vi "SDSU_ReadDACS_orig.vi"(7 "fd":i32, 8 "error in (no error)":errorcluster, 9 "argument":string, 10 "action":T1(ring), 11 "file path":path=path "/home/arcconfig/DHE_DACS.cfg") -> (0 "error out":errorcluster, 1 "response":string, 2 "Table":string[][](table), 3 "file path out":path=path "/home/ArcVIEW/ConfigFiles/PI_laboratory.cfg", 5 "index":i32, 6 "fd out":i32)   [LabVIEW 2016]
panel:
  out "resolutions":string[][](array[string])
  in  "current index":u8=6
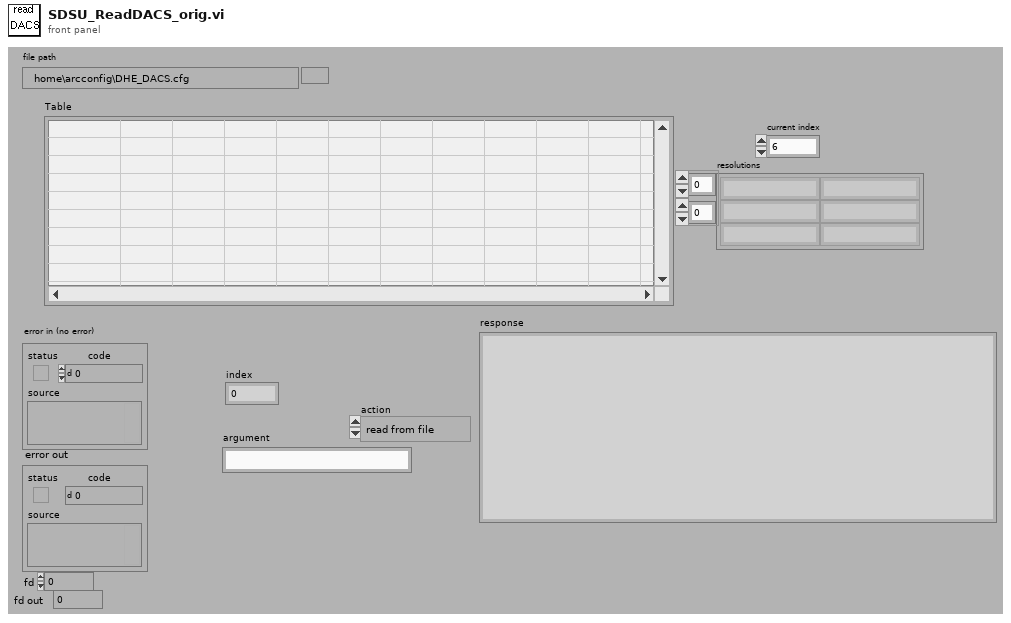
[diagram p1: front panel]
types:
  T1 = enum16{"read from file", "find", "set", "set_to_default", "get all"}
  T2 = typedef "DatabaseHand_RefNum.ctl" = refnum<vi>
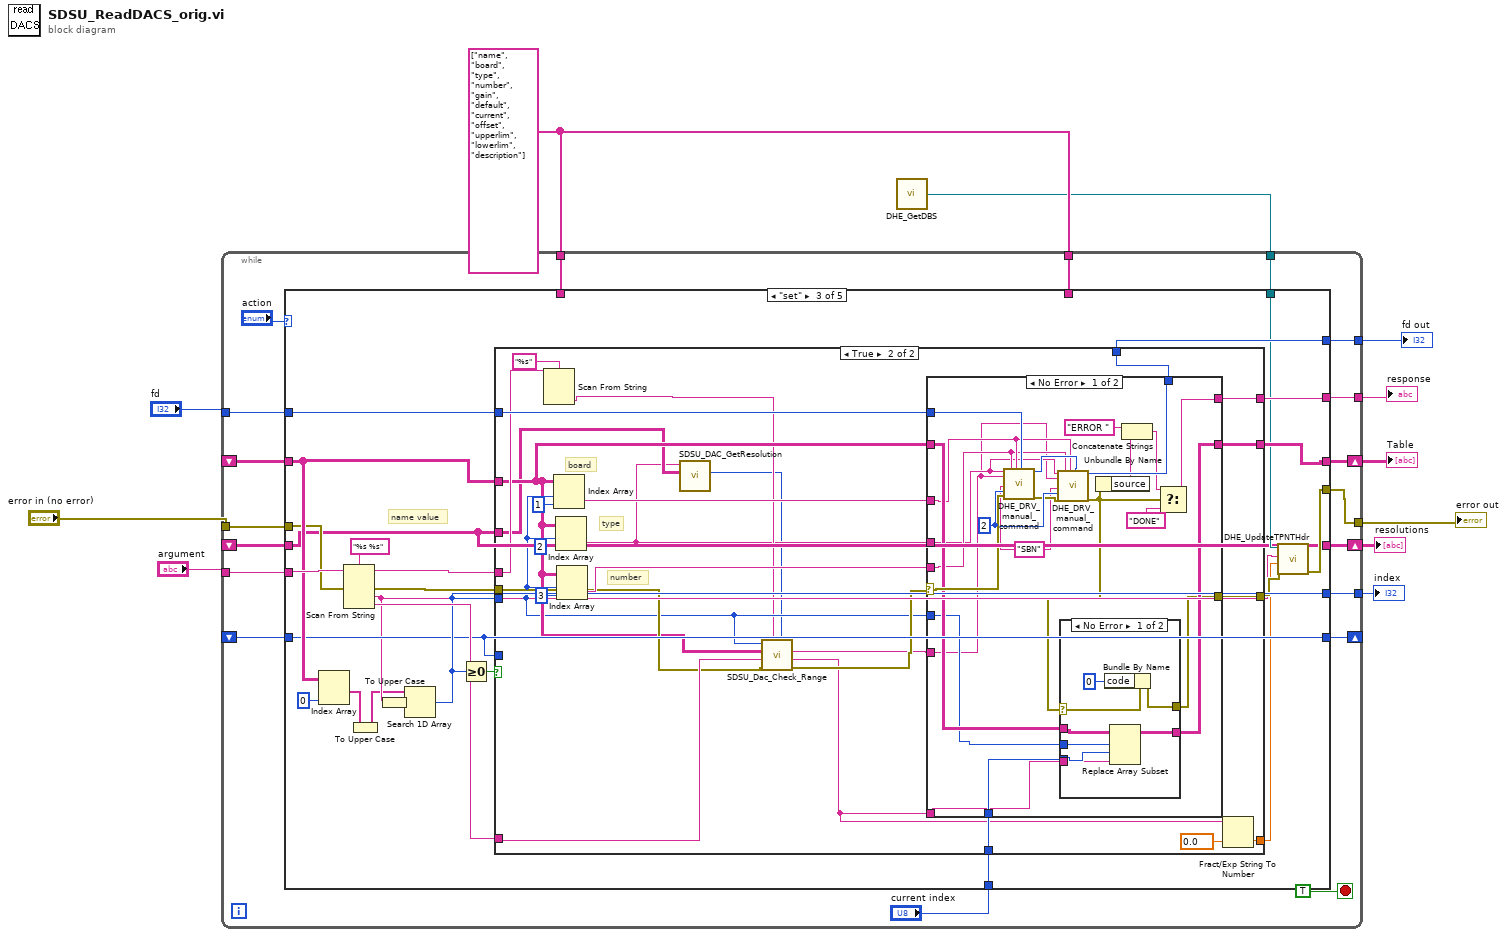
[diagram p0: block diagram]
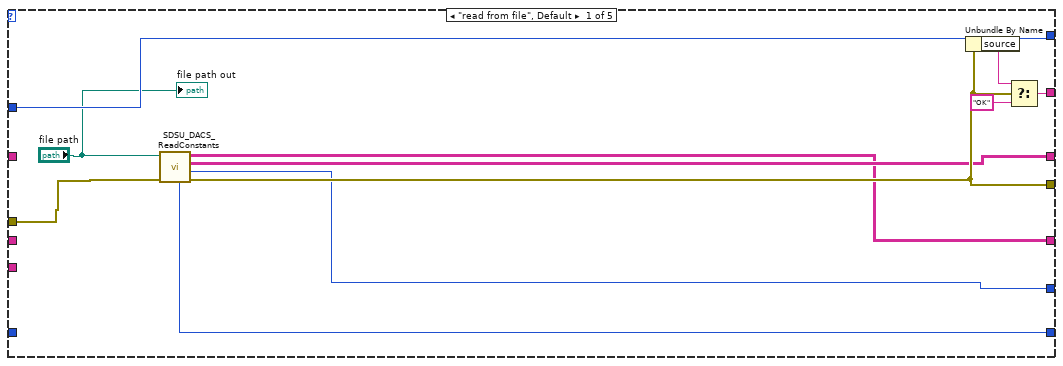
[diagram p2: hidden frame]
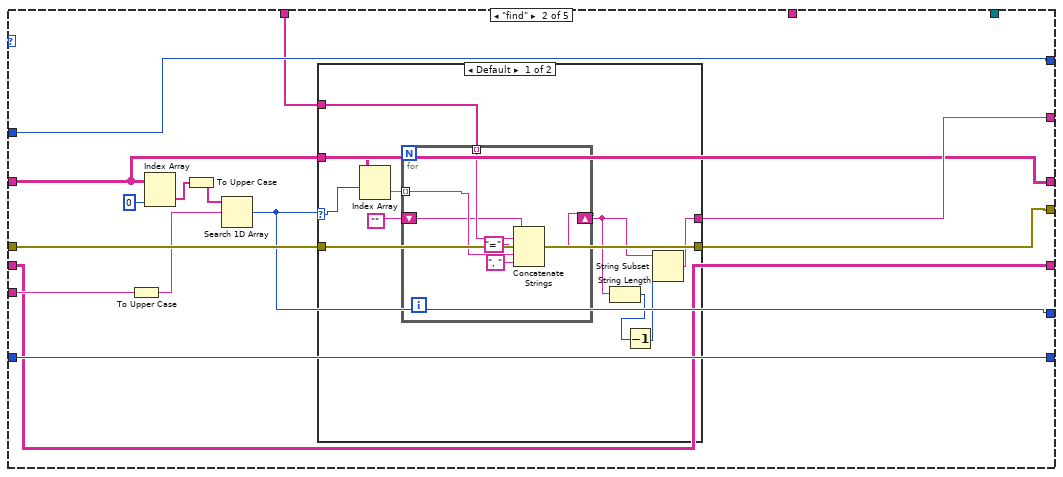
[diagram p3: hidden frame]
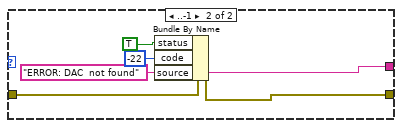
[diagram p4: hidden frame]
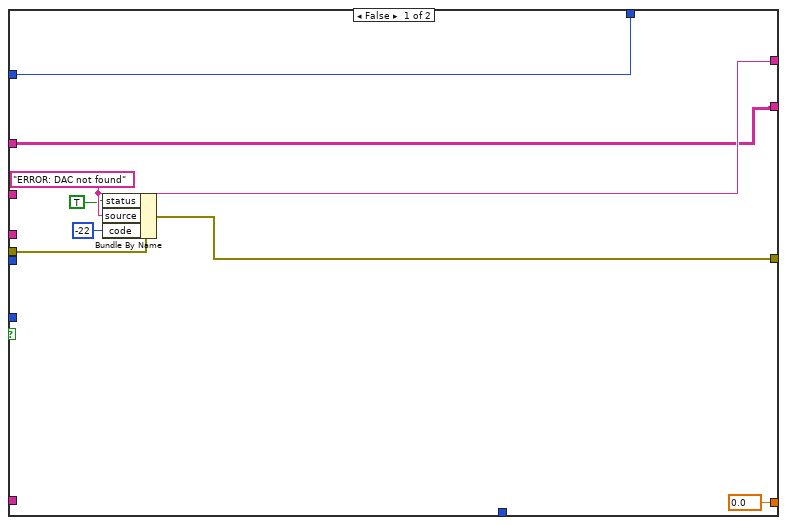
[diagram p5: hidden frame]
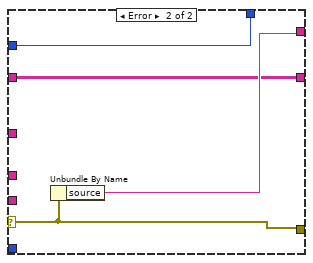
[diagram p7: hidden frame]
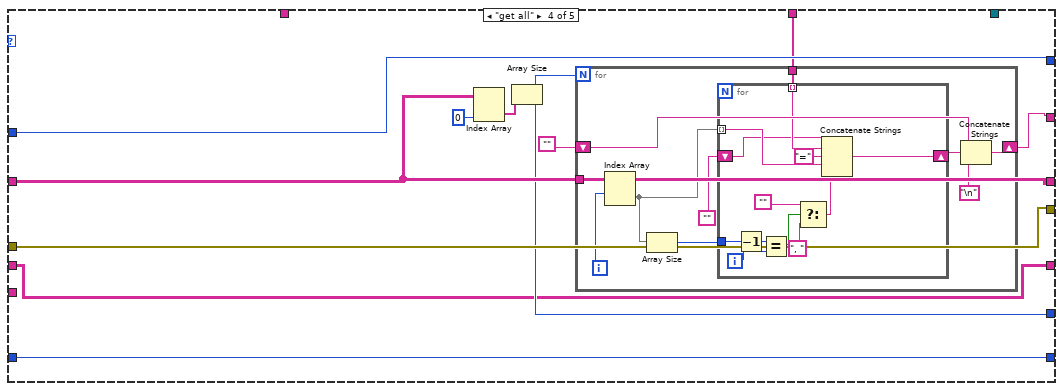
[diagram p8: hidden frame]
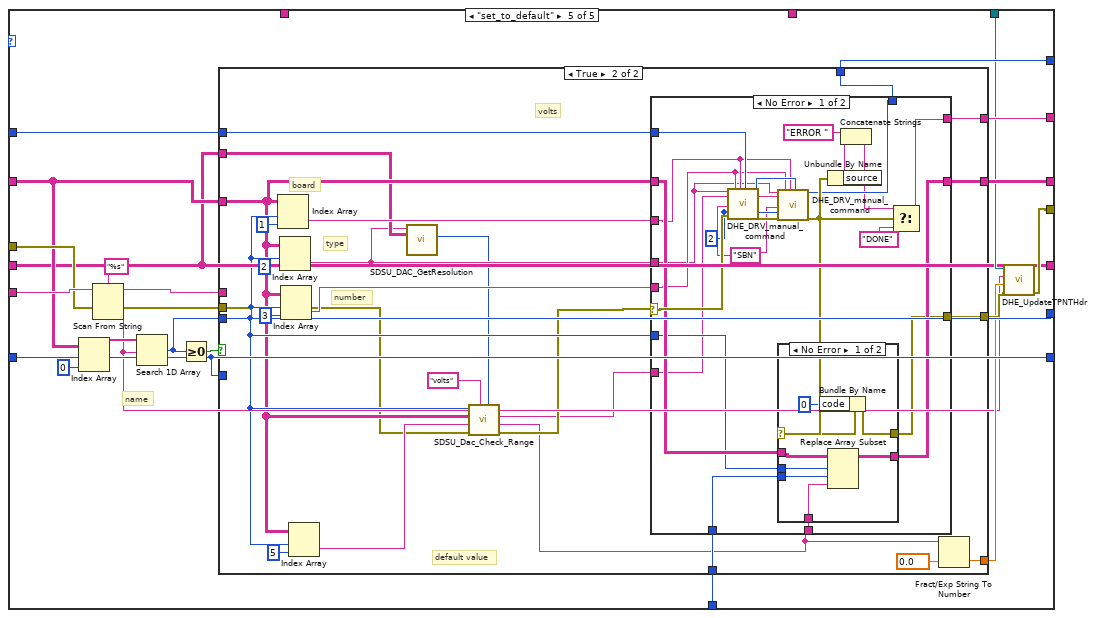
[diagram p9: hidden frame]
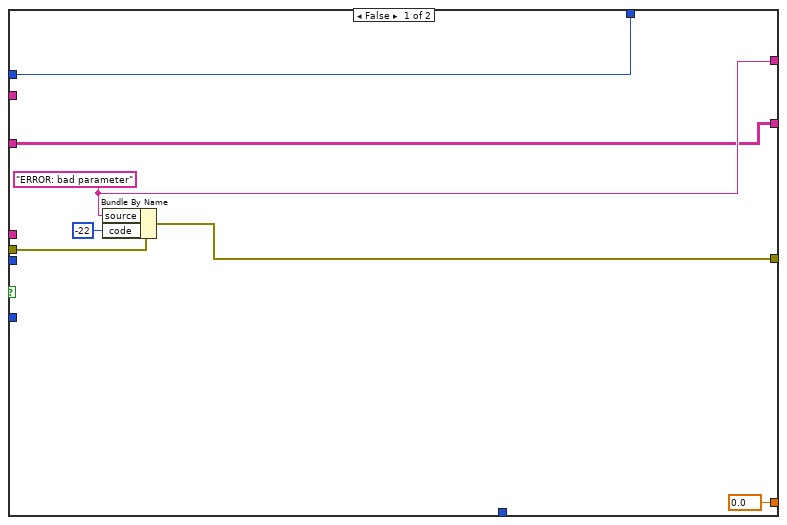
[diagram p10: hidden frame]
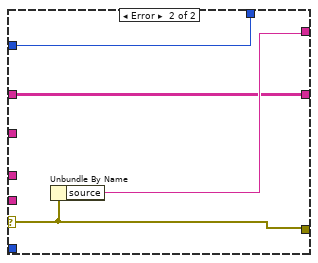
[diagram p12: hidden frame]
diagram:
  w4 = string[] ["name", "board", "type", "number", "gain", "default", "current", "offset", "upperlim", "lowerlim", "description"]
  n1 = call "DHE_GetDBS.vi"() -> ("DHE_DBSRef"=w2:T2)  [unwired: 9 out]
  n2 = while {
    shift-right: [w29] -> w10
    shift-left: _ -> [w25]
    tunnel: "error in (no error)" -> [w28]
    tunnel: [w27] -> w3
    tunnel: [w24] -> w9
    tunnel: "argument" -> [w23]
    tunnel: "fd" -> [w22]
    tunnel: [w21] -> w6
    tunnel: [w18] -> w5
    tunnel: w4 -> [w20]
    tunnel: w4 -> [w19]
    shift-right: [w16] -> _
    shift-left: _ -> [w15]
    tunnel: w2 -> [w14]
    shift-right: [w13] -> w1
    shift-left: _ -> [w12]
    stop <- TRUE stop-if-true
    n3 = case shown="\"set\"" "action" {
      tunnel: [w34 w50 w88 w177 w214] -> w29
      tunnel: w28 -> [w37 w53 w91 w178 w224]
      tunnel: [w35 w52 w84 w178 w209] -> w27
      tunnel: w25 -> [_ w50 w93 w177 w213]
      tunnel: [w39 w51 w94 w175 w220] -> w24
      tunnel: w23 -> [_ w54 w100 _ w226]
      tunnel: w22 -> [w38 w49 w97 w180 w222]
      tunnel: [w38 w49 w96 w180 w221] -> w21
      tunnel: w20 -> [_ w48 _ _ _]
      tunnel: w19 -> [_ _ _ w179 _]
      tunnel: [w33 w47 w89 w174 w215] -> w18
      tunnel: "current index" -> [_ _ w87 _ w212]
      tunnel: [w32 w46 w86 w173 w211] -> w16
      tunnel: w15 -> [_ w46 w86 w173 w211]
      tunnel: w14 -> [_ _ w81 _ w208]
      tunnel: [w31 w45 w80 w172 w205] -> w13
      tunnel: w12 -> [_ w45 w80 w172 w205]
      frame "read from file", Default {
        n4 = call "SDSU_DACS_ReadConstants.vi"("error in (no error)"=w37, "file path"="file path") -> ("error out"=w35:errorcluster, "number of dacs"=w33:i32, "constants"=w34:string[][], "resolutions"=w31:string[][], "resolution"=w32:i32)  [unwired: 5 out]
        n5 = Unbundle By Name(w35) -> ("source"=w41:string)
        n6 = Select(t=w41, s=w35, f="OK") -> (s? t:f=w39:string)
        "file path out" <- "file path"
      }
      frame "find" {
        n7 = To Upper Case(1:w54) -> (0:w42:string)
        n8 = Index Array(array=w50, index (col)=0 ("disabled index (col)")) -> (element=w44:string[])  [unwired: 1 in]
        n9 = To Upper Case(1:w44) -> (0:w43:string[])
        n10 = Search 1D Array(1D array=w43, element=w42) -> (index of element=w47:i32)  [unwired: 1 out]
        n11 = case shown="Default" w47 {
          selector: w47 -> [w63 _]
          tunnel: w50 -> [w64 _]
          tunnel: w53 -> [w65 w76]
          tunnel: [w65 w75] -> w52
          tunnel: w48 -> [w61 _]
          tunnel: [w57 w72] -> w51
          frame Default {
            n12 = Index Array(array=w64, index (row)=w63) -> (element=w62:string[])  [unwired: 1 in]
            n13 = for {
              tunnel: w62 -> [w71] mode=indexing
              tunnel: w61 -> [w70] mode=indexing
              shift-right: [w69] -> w58
              shift-left: "" -> [w68]
              n14 = Concatenate Strings(w68, w70, "=" ("string"), w71, ", " ("string")) -> (w69:string)
            }
            n15 = String Length(string=w58) -> (length=w59:i32)
            n16 = Decrement(x=w59) -> (x-1=w56:i32)
            n17 = String Subset(string=w58, length (rest)=w56) -> (substring=w57:string)  [unwired: 1 out]
          }
          frame ..-1 {
            w72 = "ERROR: DAC  not found" ("source")
            n18 = Bundle By Name(cluster=w76, "status"=TRUE, "code"=-22, "source"=w72) -> (w75:errorcluster)
          }
        }
      }
      frame "set" {
        # "name value"
        n19 = Index Array(array=w93, index (col)=0 ("disabled index (col)")) -> (element=w79:string[])  [unwired: 1 in]
        n20 = Scan From String(format string="%s %s", input string=w100, error in=w91) -> (remaining string=w98:string, output 1=w83:string, output 2=w95:string)  [unwired: 1 in, 4 out]
        n21 = To Upper Case(1:w79) -> (0:w78:string[])
        n22 = To Upper Case(1:w83) -> (0:w77:string)
        n23 = Search 1D Array(1D array=w78, element=w77) -> (index of element=w89:i32)  [unwired: 1 out]
        n24 = Greater Or Equal To 0?(x=w89) -> (x >= 0?=w90:bool)
        n25 = case shown="True" w90 {
          tunnel: [w107 w129] -> w85
          tunnel: w89 -> [_ w116]
          tunnel: w98 -> [_ w127]
          tunnel: w93 -> [w103 w117]
          tunnel: w97 -> [w106 w134]
          tunnel: [w106 w133] -> w96
          tunnel: w95 -> [_ w121]
          tunnel: [w105 w128] -> w94
          tunnel: w91 -> [w104 w120]
          tunnel: [w103 w123] -> w88
          tunnel: w87 -> [_ w122]
          tunnel: w86 -> [_ _]
          tunnel: [0.0 w113] -> w82
          tunnel: w80 -> [_ w111]
          frame False {
            w105 = "ERROR: DAC not found" ("source")
            n26 = Bundle By Name(cluster=w104, "status"=TRUE, "source"=w105, "code"=-22) -> (w107:errorcluster)
          }
          frame True {
            # "number"
            # "type"
            # "board"
            n27 = Scan From String(format string="%s", input string=w127) -> (output 1=w115:string)  [unwired: 2 in, 4 out]
            n28 = Index Array(array=w117, index (row)=w116, index (col)=1 ("disabled index (col)")) -> (element=w125:string)
            n29 = Index Array(array=w117, index (row)=w116, index (col)=2 ("disabled index (col)")) -> (element=w110:string)
            n30 = Index Array(array=w117, index (row)=w116, index (col)=3 ("disabled index (col)")) -> (element=w124:string)
            n31 = call "SDSU_DAC_GetResolution.vi"("resolutions"=w111, "type"=w110) -> ("max counts"=w109:i32)  [unwired: 9 out]
            n32 = call "SDSU_Dac_Check_Range.vi"("resolution"=w109, "unit"=w115, "error in (no error)"=w120, "value in"=w121, "DACS"=w117, "dac number"=w116) -> ("error out"=w119:errorcluster, "volts value"=w114:string, "dac value"=w118:string)  [unwired: 3 out]
            n33 = case shown="No Error" w119 {
              selector: w119 -> [w154 w170]
              tunnel: w134 -> [w157 w171]
              tunnel: [w144 w171] -> w133
              tunnel: [w147 w170] -> w129
              tunnel: [w155 w169] -> w128
              tunnel: w110 -> [w139 _]
              tunnel: w125 -> [w141 _]
              tunnel: w124 -> [w140 _]
              tunnel: w118 -> [w135 _]
              tunnel: w117 -> [w152 w168]
              tunnel: [w149 w168] -> w123
              tunnel: w116 -> [w151 _]
              tunnel: w122 -> [w150 _]
              tunnel: w114 -> [w148 _]
              frame No Error {
                w153 = i16 2 ("short board_dest")
                w142 = "SBN" ("command")
                n34 = call "DHE_DRV_manual_command.vi"("arg3"=w139, "arg4"=w135, "command"=w142, "short board_dest"=w153, "error in (no error)"=w154, "arg2"=w140, "arg1"=w141, "fd"=w157) -> ("fd"=w145:i32, "error out"=w146:errorcluster)  [unwired: 1 in, 9 out]
                n35 = call "DHE_DRV_manual_command.vi"("arg3"=w139, "arg4"=w135, "command"=w142, "short board_dest"=w153, "error in (no error)"=w146, "arg2"=w140, "arg1"=w141, "fd"=w145) -> ("fd"=w144:i32, "error out"=w143:errorcluster)  [unwired: 1 in, 9 out]
                n36 = case shown="No Error" w143 {
                  selector: w143 -> [w159 w166]
                  tunnel: w152 -> [w165 w167]
                  tunnel: w151 -> [w164 _]
                  tunnel: w150 -> [w163 _]
                  tunnel: [w162 w167] -> w149
                  tunnel: w148 -> [w161 _]
                  tunnel: [w158 w166] -> w147
                  frame No Error {
                    n37 = Bundle By Name(cluster=w159, "code"=0) -> (w158:errorcluster)
                    n38 = Replace Array Subset(array=w165, new element=w161, index (row)=w164, index (col)=w163) -> (w162:string[][])
                  }
                  frame Error {
                  }
                }
                n39 = Unbundle By Name(w143) -> ("source"=w136:string)
                n40 = Concatenate Strings("ERROR " ("string"), w136) -> (w137:string)
                n41 = Select(t=w137, s=w143, f="DONE") -> (s? t:f=w155:string)
              }
              frame Error {
                n42 = Unbundle By Name(w170) -> ("source"=w169:string)
              }
            }
            n43 = Fract/Exp String To Number(string=w114, default (0 dbl)=0.0) -> (number=w113:dbl)  [unwired: 3 out]
          }
        }
        n44 = call "DHE_UpdateTPNTHdr.vi"("error in (no error)"=w85, "TP value"=w82, "TP name"=w83, "Database RefNum in"=w81) -> ("error out"=w84:errorcluster)  [unwired: 7 out]
      }
      frame "get all" {
        n45 = Index Array(array=w177, index (col)=0 ("disabled index (col)")) -> (element=w181:string[])  [unwired: 1 in]
        n46 = Array Size(array=w181) -> (size(s)=w174:i32)
        n47 = for {
          N: w174 -> [_]
          tunnel: w179 -> [w192]
          tunnel: w177 -> [w191]
          shift-right: [w188] -> w175
          shift-left: "" -> [w187]
          i -> [w190]
          n48 = Index Array(array=w191, index (row)=w190) -> (element=w185:string[])  [unwired: 1 in]
          n49 = Array Size(array=w185) -> (size(s)=w184:i32)
          n50 = for {
            tunnel: w185 -> [w202] mode=indexing
            tunnel: w192 -> [w204] mode=indexing
            shift-right: [w194] -> w183
            shift-left: "" -> [w201]
            tunnel: w184 -> [w199]
            i -> [w200]
            n51 = Decrement(x=w199) -> (x-1=w193:i32)
            n52 = Equal?(x=w193, y=w200) -> (x = y?=w198:bool)
            n53 = Select(t="", s=w198, f=", ") -> (s? t:f=w196:string)
            n54 = Concatenate Strings(w201, w204, "=" ("string"), w202, w196) -> (w194:string)
          }
          n55 = Concatenate Strings(w187, w183, "\n") -> (w188:string)
        }
      }
      frame "set_to_default" {
        # "name"
        n56 = Index Array(array=w213, index (col)=0 ("disabled index (col)")) -> (element=w218:string[])  [unwired: 1 in]
        n57 = Scan From String(format string="%s", input string=w226, error in=w224) -> (remaining string=w223:string, error out=w216:errorcluster, output 1=w206:string)  [unwired: 1 in, 2 out]
        n58 = Search 1D Array(1D array=w218, element=w206) -> (index of element=w215:i32)  [unwired: 1 out]
        n59 = Greater Or Equal To 0?(x=w215) -> (x >= 0?=w217:bool)
        n60 = case shown="True" w217 {
          tunnel: [w232 w253] -> w210
          tunnel: w215 -> [_ w246]
          tunnel: w223 -> [_ _]
          tunnel: w213 -> [w228 w245]
          tunnel: w222 -> [w231 w258]
          tunnel: [w231 w257] -> w221
          tunnel: [w230 w252] -> w220
          tunnel: w216 -> [w229 w242]
          tunnel: [w228 w248] -> w214
          tunnel: w212 -> [_ w247]
          tunnel: w211 -> [_ _]
          tunnel: [0.0 w238] -> w207
          tunnel: w205 -> [_ w236]
          frame False {
            w230 = "ERROR: bad parameter" ("source")
            n61 = Bundle By Name(cluster=w229, "source"=w230, "code"=-22) -> (w232:errorcluster)
          }
          frame True {
            # "default value"
            # "volts"
            # "number"
            # "type"
            # "board"
            n62 = Index Array(array=w245, index (row)=w246, index (col)=1 ("disabled index (col)")) -> (element=w251:string)
            n63 = Index Array(array=w245, index (row)=w246, index (col)=2 ("disabled index (col)")) -> (element=w235:string)
            n64 = Index Array(array=w245, index (row)=w246, index (col)=3 ("disabled index (col)")) -> (element=w250:string)
            n65 = Index Array(array=w245, index (row)=w246, index (col)=5 ("disabled index (col)")) -> (element=w243:string)
            n66 = call "SDSU_DAC_GetResolution.vi"("resolutions"=w236, "type"=w235) -> ("max counts"=w234:i32)  [unwired: 9 out]
            n67 = call "SDSU_Dac_Check_Range.vi"("resolution"=w234, "unit"="volts", "error in (no error)"=w242, "value in"=w243, "DACS"=w245, "dac number"=w246) -> ("error out"=w241:errorcluster, "volts value"=w239:string, "dac value"=w240:string)  [unwired: 3 out]
            n68 = case shown="No Error" w241 {
              selector: w241 -> [w278 w294]
              tunnel: w258 -> [w281 w295]
              tunnel: [w268 w295] -> w257
              tunnel: [w272 w294] -> w253
              tunnel: [w279 w293] -> w252
              tunnel: w235 -> [w264 _]
              tunnel: w251 -> [w266 _]
              tunnel: w250 -> [w265 _]
              tunnel: w240 -> [w263 _]
              tunnel: w245 -> [w277 w292]
              tunnel: [w276 w292] -> w248
              tunnel: w246 -> [w275 _]
              tunnel: w247 -> [w274 _]
              tunnel: w239 -> [w273 _]
              frame No Error {
                w267 = i16 2 ("short board_dest")
                w262 = "SBN" ("command")
                n69 = call "DHE_DRV_manual_command.vi"("arg3"=w264, "arg4"=w263, "command"=w262, "short board_dest"=w267, "error in (no error)"=w278, "arg2"=w265, "arg1"=w266, "fd"=w281) -> ("fd"=w269:i32, "error out"=w271:errorcluster)  [unwired: 1 in, 9 out]
                n70 = call "DHE_DRV_manual_command.vi"("arg3"=w264, "arg4"=w263, "command"=w262, "short board_dest"=w267, "error in (no error)"=w271, "arg2"=w265, "arg1"=w266, "fd"=w269) -> ("fd"=w268:i32, "error out"=w270:errorcluster)  [unwired: 1 in, 9 out]
                n71 = case shown="No Error" w270 {
                  selector: w270 -> [w284 w290]
                  tunnel: w277 -> [w289 w291]
                  tunnel: w275 -> [w288 _]
                  tunnel: [w287 w291] -> w276
                  tunnel: w274 -> [w286 _]
                  tunnel: w273 -> [w285 _]
                  tunnel: [w283 w290] -> w272
                  frame No Error {
                    n72 = Bundle By Name(cluster=w284, "code"=0) -> (w283:errorcluster)
                    n73 = Replace Array Subset(array=w289, new element=w285, index (row)=w288, index (col)=w286) -> (w287:string[][])
                  }
                  frame Error {
                  }
                }
                n74 = Unbundle By Name(w270) -> ("source"=w260:string)
                n75 = Concatenate Strings("ERROR " ("string"), w260) -> (w259:string)
                n76 = Select(t=w259, s=w270, f="DONE") -> (s? t:f=w279:string)
              }
              frame Error {
                n77 = Unbundle By Name(w294) -> ("source"=w293:string)
              }
            }
            n78 = Fract/Exp String To Number(string=w239, default (0 dbl)=0.0) -> (number=w238:dbl)  [unwired: 3 out]
          }
        }
        n79 = call "DHE_UpdateTPNTHdr.vi"("error in (no error)"=w210, "TP value"=w207, "TP name"=w206, "Database RefNum in"=w208) -> ("error out"=w209:errorcluster)  [unwired: 7 out]
      }
    }
  }
  "error out" <- w3
  "Table" <- w10
  "response" <- w9
  "fd out" <- w6
  "index" <- w5
  "resolutions" <- w1
